vi "Downsample Physical Image.vi"(7 "Reduction Factor":i32=4, 8 "error in":errorcluster, 11 "Physical Image In":T1) -> (0 "error out":errorcluster, 3 "Physical Image Out":T1)   [LabVIEW 2023]
uses:
  Type Definitions/Physical Image.ctl
  Vec3d Class/Vec3d.lvclass
  <vilib>/vision/Image Controls.llb/IMAQ Image.ctl
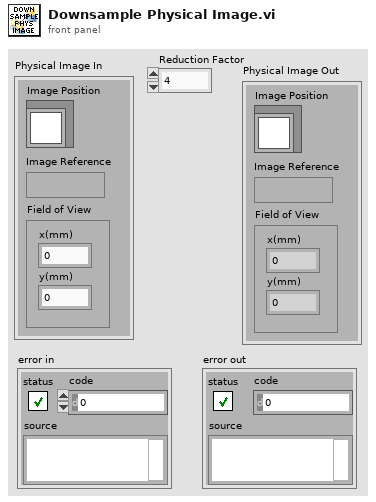
[diagram p1: front panel]
types:
  T1 = typedef "Physical Image.ctl" = cluster{"Image Position":refnum<class "Vec3d.lvclass">, "Image Reference":T2, "Field of View":cluster{"x(mm)":dbl, "y(mm)":dbl}}
  T2 = typedef "IMAQ Image.ctl" = refnum<image>
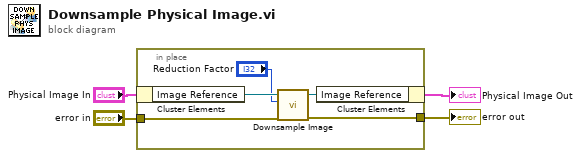
[diagram p0: block diagram]
diagram:
  n1 = in-place {
    in-place-border: "error in" -> [w8]
    in-place-border: [w5] -> w3
    n2 = in-place-cluster #1("Physical Image In") -> ("Image Reference"=w9:T2)
    n3 = call "Downsample Image.vi"("error in"=w8, "Reduction Factor"="Reduction Factor", "Refnum in"=w9) -> ("error out"=w5:errorcluster, "Refnum out"=w6:T2)  [unwired: 7 in]
    n4 = in-place-cluster #1("Image Reference"=w6) -> (→"Physical Image Out":T1)
  }
  "error out" <- w3
